vi "S2C_ErrorPrompt.vi"(8 "Error In":errorcluster, 11 "ErrMsgIn":string) -> (0 "Error Out":errorcluster)   [LabVIEW 2024]
doc: "Generic error prompt designed to display error information to the user."
panel:
  out "Init":bool
  in  "Ack":bool
  out "ErrMsg":string caption="Error Message"
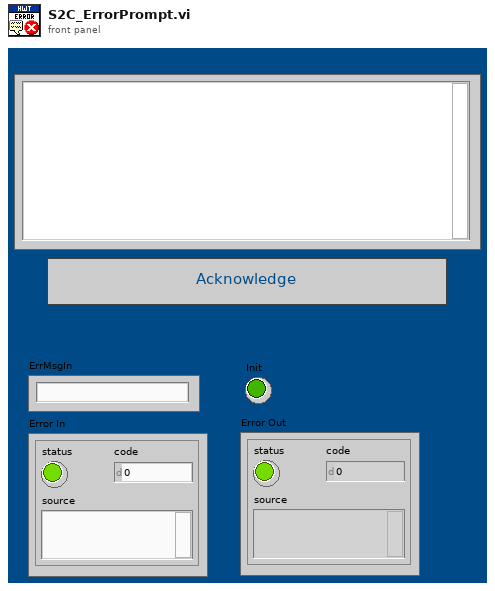
[diagram p1: front panel]
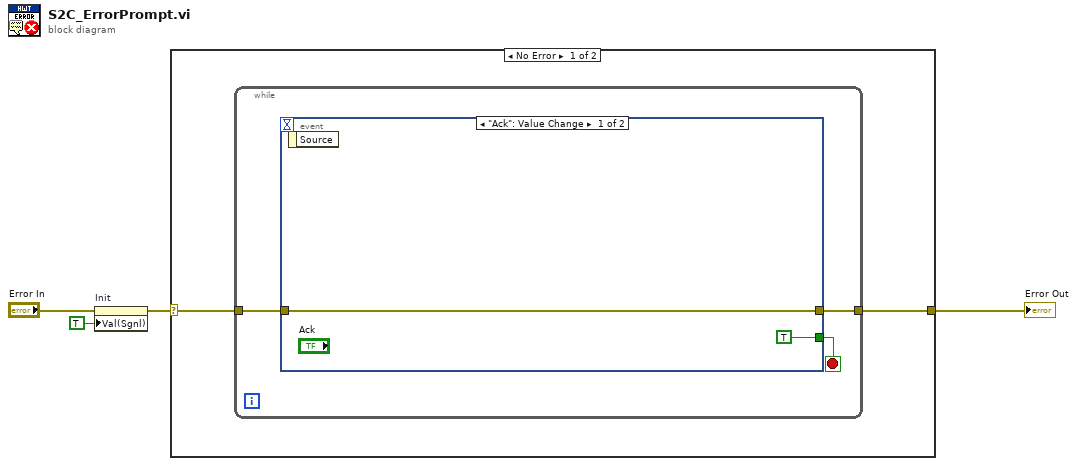
[diagram p0: block diagram]
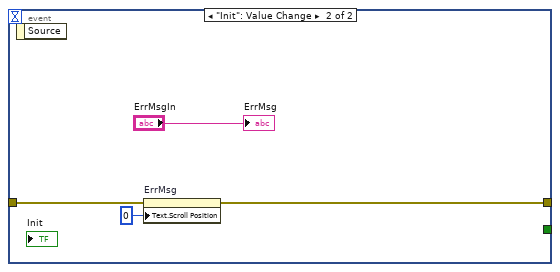
[diagram p2: hidden frame]
diagram:
  n1 = property on="Init" class="Bool (strict)"(error in="Error In", "Val(Sgnl)"=TRUE ("Value (Signaling)")) -> (error out=w2:errorcluster)  [unwired: 1 in, 1 out]
  n2 = case shown="No Error" w2 {
    selector: w2 -> [w6 w16]
    tunnel: [w5 w16] -> w4
    frame No Error {
      n3 = while {
        tunnel: w6 -> [w9]
        tunnel: [w8] -> w5
        stop <- w7 stop-if-true
        n4 = event shown="[0] \"Ack\": Value Change" {
          selector: _ -> [_ _]
          dyn-events: _ -> [_ _]
          timeout: _ -> [_ _]
          tunnel: w9 -> [w11 w14]
          tunnel: [w11 w12] -> w8
          tunnel: [TRUE _] -> w7
          event "Ack": Value Change {
            n5 = event-data() -> ()  [unwired: 1 in, 1 out]
          }
          event "Init": Value Change {
            n6 = event-data() -> ()  [unwired: 1 in, 1 out]
            n7 = property on="ErrMsg" class="Str"(error in=w14, "Text.Scroll Position"=u32 0) -> (error out=w12:errorcluster)  [unwired: 1 in, 1 out]
            "ErrMsg" <- "ErrMsgIn"
          }
        }
      }
    }
    frame Error {
    }
  }
  "Error Out" <- w4
